vi "240126_Keyboard_TEST.vi"() -> ()   [LabVIEW 2014]
uses:
  <vilib>/event_ctls.llb/eventvkey.ctl
panel:
  out "String":string
  out "VKey":T1
  out "ScanCode":i16
  in  "stop":bool
  out "PlatMods":T2
  out "Char":i16
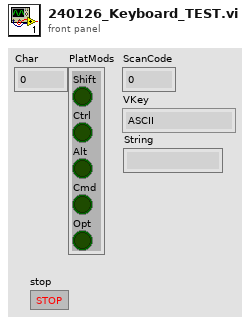
[diagram p1: front panel]
types:
  T1 = typedef "eventvkey.ctl" = enum16{"ASCII", "Enter", "Return", "Shift", "Ctrl", "Alt", "Cmd", "Opt", "Caps", "NumLock", "Clear", "Break", "Up", "Down", "Left", "Right", "Insert", "Delete", "Home", "End", "PageUp", "PageDown", "Escape", "Help", "Pause", "ScrollLock", "F1", "F2", "F3", "F4", "F5", "F6", "F7", "F8", "F9", "F10", "F11", "F12", "F13", "F14", "F15", "F16", "F17", "F18", "F19", "F20", "F21", "F22", "F23", "F24", "Play", "VolumeUp", "VolumeDown", "Mute", "Two Byte Char"}
  T2 = cluster{"Shift":bool, "Ctrl":bool, "Alt":bool, "Cmd":bool, "Opt":bool}
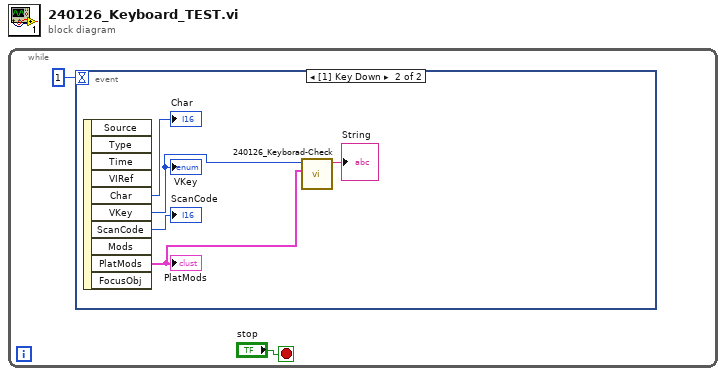
[diagram p0: block diagram]
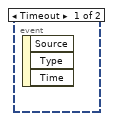
[diagram p2: hidden frame]
diagram:
  n1 = while {
    stop <- "stop" stop-if-true
    n2 = event shown="[1] Key Down" {
      selector: _ -> [_ _]
      dyn-events: _ -> [_ _]
      timeout: 1 -> [_ _]
      event Timeout {
        n3 = event-data() -> ()  [unwired: 1 in, 3 out]
      }
      event Key Down {
        n4 = event-data() -> ("Char"=→"Char":i16, "VKey"=w5:T1, "ScanCode"=→"ScanCode":i16, "PlatMods"=w4:T2)  [unwired: 1 in, 6 out]
        "PlatMods" <- w4
        "VKey" <- w5
        n5 = call "240126_Keyborad-Check.vi"("PlatMods"=w4, "VKey"=w5) -> ("String"=→"String":string)  [unwired: 8 in, 1 out]
      }
    }
  }
